vi "Set AccessType.vi"(8 "error in":errorcluster, 10 "Value":refnum<class "Value.lvclass">, 11 "Object Type in":refnum<class "ARRAY.lvclass">) -> (0 "error out":errorcluster, 3 "Object Type out":refnum<class "ARRAY.lvclass">)   [LabVIEW 2024, in "Electronic Datasheet.lvlib" / "ARRAY.lvclass"]
uses:
  ARRAY.lvclass
  Value/Value.lvclass
  Electronic Datasheet.lvlib
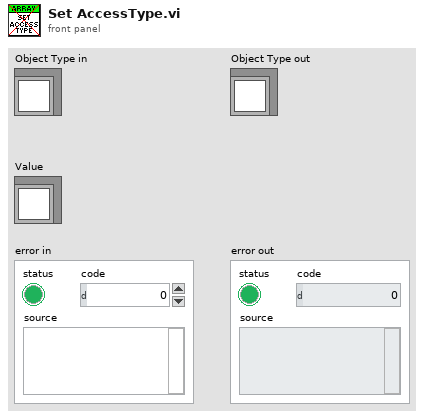
[diagram p1: front panel]
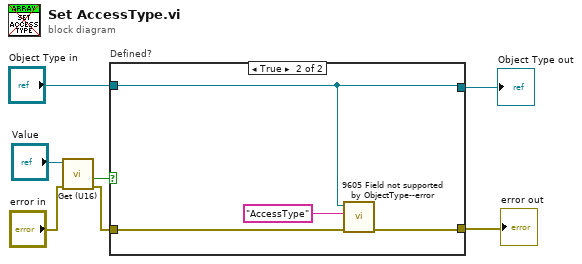
[diagram p0: block diagram]
diagram:
  n1 = call "Get (U16).vi"("error in"="error in", "Value in"="Value") -> ("error out"=w2:errorcluster, "Defined?"=w1:bool)  [unwired: 6 in, 2 out]
  n2 = case "Defined?" shown="True" w1 {
    tunnel: [w9 w12] -> w5
    tunnel: "Object Type in" -> [w8 w10]
    tunnel: [w8 w10] -> w6
    tunnel: w2 -> [w9 w13]
    frame False {
    }
    frame True {
      n3 = call "9605 Field not supported by ObjectType--error.vi"("error in"=w13, "Field Name"="AccessType" ("Field name"), "Object Type Base"=w10) -> ("error out"=w12:errorcluster)  [unwired: 8 in]
    }
  }
  "Object Type out" <- w6
  "error out" <- w5
